vi "CaliperEntrySetToNone.vi"(8 "error in (no error)":errorcluster, 11 "CaliperEntryList":T1[](array[typedef]) {"CaliperType" items=["Distance", "Mid Point", "Perpendicular Projection", "Lines Intersection", "Angle from Horizontal", "Angle from Vertical", "Angle Defined by 3 Points", "Angle Defined by 4 Points", "Bissecting Line", "Mid Line", "Center of Mass", "Area", "Line Fit", "Circle Fit", "Ellipse Fit"]}) -> (0 "error out":errorcluster, 3 "CaliperEntryOut":T1[](array[typedef]) {"CaliperType" items=["Distance", "Mid Point", "Perpendicular Projection", "Lines Intersection", "Angle from Horizontal", "Angle from Vertical", "Angle Defined by 3 Points", "Angle Defined by 4 Points", "Bissecting Line", "Mid Line", "Center of Mass", "Area", "Line Fit", "Circle Fit", "Ellipse Fit"]})   [LabVIEW 2019]
uses:
  Controls/CaliperDataEntry.ctl
  Controls/CaliperType.ctl
  Controls/SelectionListEntry.ctl
  Controls/SelectionListEntryPointType.ctl
  Controls/CaliperResult.ctl
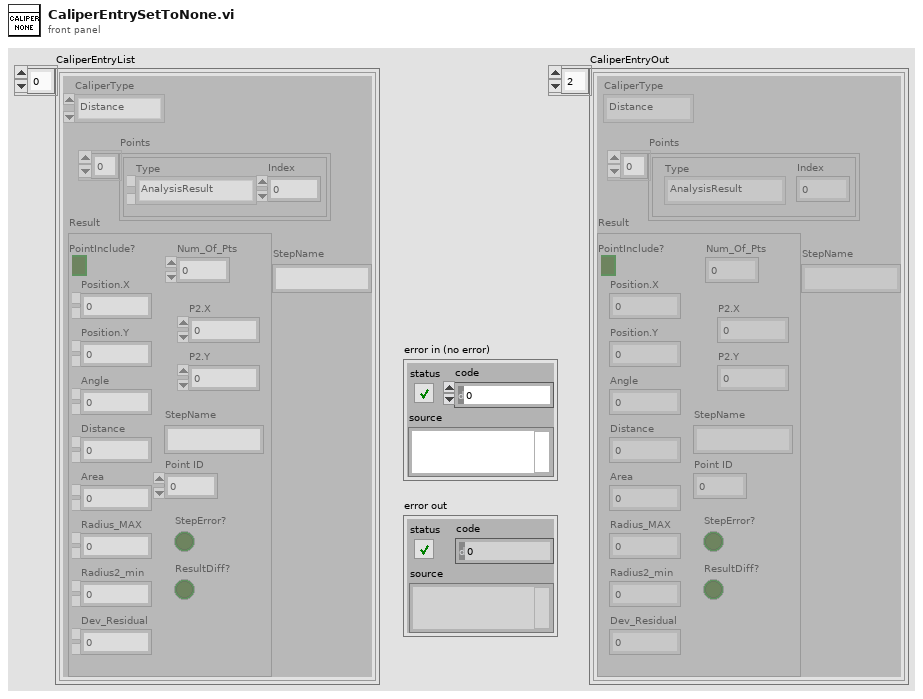
[diagram p1: front panel]
types:
  T1 = typedef "CaliperDataEntry.ctl" = cluster{"CaliperType":T2, "Points":T3[], "Result":T5, "StepName":string}
  T2 = typedef "CaliperType.ctl" = u32
  T3 = typedef "SelectionListEntry.ctl" = cluster{"Type":T4, "Index":i32}
  T4 = typedef "SelectionListEntryPointType.ctl" = enum16{"AnalysisResult", "CaliperResult"}
  T5 = typedef "CaliperResult.ctl" = cluster{"PointInclude?":bool, "Num_Of_Pts":u8, "Position.X":dbl, "Position.Y":dbl, "Angle":dbl, "Distance":dbl, "Area":dbl, "Radius_MAX":dbl, "Radius2_min":dbl, "Dev_Residual":dbl, "P2.X":dbl, "P2.Y":dbl, "StepName":string, "Point ID":u8, "StepError?":bool, "ResultDiff?":bool}
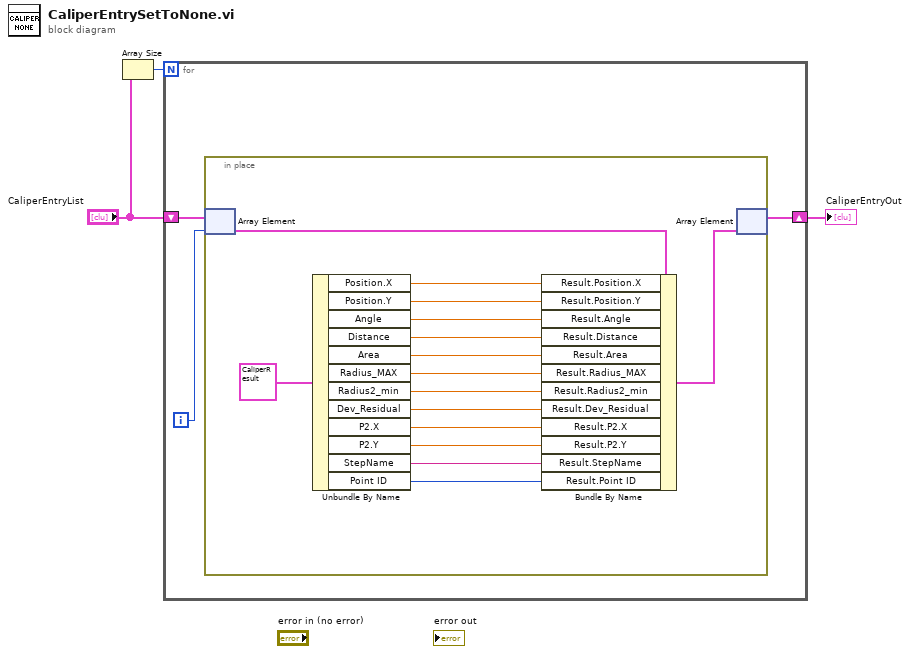
[diagram p0: block diagram]
diagram:
  n1 = Array Size(array="CaliperEntryList") -> (size(s)=w2:i32)
  n2 = for {
    N: w2 -> [_]
    shift-right: [w4] -> w3
    shift-left: "CaliperEntryList" -> [w6]
    i -> [w5]
    n3 = in-place {
      n4 = in-place-array #1(w6, w5) -> (w21:T1)
      n5 = Unbundle By Name(T5 {"PointInclude?"=FALSE, "Num_Of_Pts"=0, "Position.X"=0.0, "Position.Y"=0.0, "Angle"=0.0, "Distance"=0.0, "Area"=0.0, "Radius_MAX"=0.0, "Radius2_min"=0.0, "Dev_Residual"=0.0, "P2.X"=0.0, "P2.Y"=0.0, "StepName"="", "Point ID"=0, "StepError?"=FALSE, "ResultDiff?"=FALSE} ("Result")) -> ("Position.X"=w18:dbl, "Position.Y"=w17:dbl, "Angle"=w16:dbl, "Distance"=w15:dbl, "Area"=w14:dbl, "Radius_MAX"=w13:dbl, "Radius2_min"=w12:dbl, "Dev_Residual"=w11:dbl, "P2.X"=w10:dbl, "P2.Y"=w9:dbl, "StepName"=w8:string, "Point ID"=w7:u8)
      n6 = Bundle By Name(cluster=w21, "Result.Position.X"=w18, "Result.Position.Y"=w17, "Result.Angle"=w16, "Result.Distance"=w15, "Result.Area"=w14, "Result.Radius_MAX"=w13, "Result.Radius2_min"=w12, "Result.Dev_Residual"=w11, "Result.P2.X"=w10, "Result.P2.Y"=w9, "Result.StepName"=w8, "Result.Point ID"=w7) -> (w20:T1)
      n7 = in-place-array #1(w20) -> (w4:T1[])  [unwired: 1 out]
    }
  }
  "CaliperEntryOut" <- w3
